vi "Set SPAN Component.vi"(7 "Protocol_only":bool, 8 "error in (no error)":errorcluster caption="Fehler (Eingang, kein Fehler)", 9 "Gasnummer":T3 min=1 max=5, 10 "Autolin Hovacal (alt)":refnum<vi>, 11 "Daten Hovacal (alt)":refnum<vi>) -> (0 "error out":errorcluster caption="Fehler (Ausgang)", 1 "Gaskomponente":T2, 2 "LogInfo-Einstellung-Cluster":T1, 3 "Komponente":string, 4 "Einheit in String":string)   [LabVIEW 2020, in "Linearisierung v2.lvlib" / "SpanEinstellungen.lvlib"]
uses:
  SpanEinstellungen.lvlib
  Gasnumber.ctl
  Visualisierungs Elemente/Auswahlfeld.ctl
  Seiten/FT-IR/FGV FT-IR Gasliste Aktionen.ctl
  Aktion Lin Daten aufarbeiten.ctl
  Gasteiler/Aktionen FGV Gasteiler Daten.ctl
  Linearisierung v2.lvlib
  Seiten/FT-IR/FT-IR.lvlib
  Gasteiler/Gasteiler.lvlib
  Gasteiler/HovaCal/Aktion_FGV_Betriebsdaten.ctl
  Gasteiler/HovaCal/HovaCal.lvlib
  Gasteiler/HovaCAL_Interface/Kommunikation/Kommunikation.lvlib
  Gasteiler/HovaCAL_Interface/Helper/Helper.lvlib
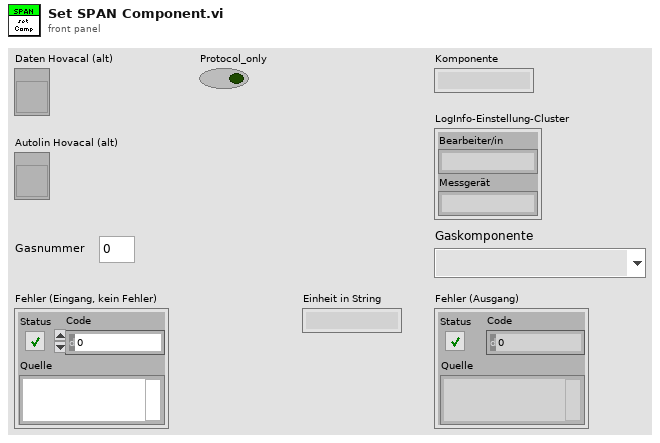
[diagram p1: front panel]
types:
  T1 = cluster{"Bearbeiter/in":string, "Messgerät":string}
  T2 = typedef "Auswahlfeld.ctl" = u16
  T3 = typedef "Linearisierung v2.lvlib/Gasnumber.ctl" = u8
  T4 = typedef "Linearisierung v2.lvlib/Gasteiler.lvlib/Aktionen FGV Gasteiler Daten.ctl" = enum16{"lesen", "Gasteiler Daten", "Seriellen Param.", "MB-Endwert", "laden", "speichern", "Anforderung", "TCP", "Aufzeichnung Start"}
  T5 = typedef "Linearisierung v2.lvlib/Aktion Lin Daten aufarbeiten.ctl" = enum16{"lesen", "Protkolldaten", "speichern", "laden", "EPA auswerten", "Tabelle schreiben", "Lin auswerten", "Tab init", "Stufentabelle", "EPA aktiviert", "Nachbehandlung laden", "Tabelle löschen", "Istwerte löschen", "Zeile löschen", "Zeile einfügen", "LIN aktiviert", "LIN/EPA aktiv laden", "EGAK Tab", "LIN übernehmen", "Tab init ohne Stufen"}
  T6 = typedef "FT-IR.lvlib/FGV FT-IR Gasliste Aktionen.ctl" = enum16{"lesen", "Gasliste FT-IR", "Gasliste ausgelesen", "laden", "speichern", "löschen"}
  T7 = typedef "Linearisierung v2.lvlib/Lin-Polynom Daten.ctl" = cluster{"Messgerät":string, "Kalibrator (Gasteiler)":string, "Bearbeiter/in":string, "Komponente":string, "Zeitstempel":timestamp, "F_max gefordert (%)":sgl, "F_max in %":sgl, "F_max in ppm":sgl, "Vorschlag Ordnung":i32, "Polynom OK":bool, "Polynomkoeff.":dbl[], "Prüfgas Konzentration":dbl, "Pfad EPA":string, "Pfad_LIN":string, "Gasnummer:":u8, "Komponentenauswahl":T8, "Verdünnungsgas":T9, "Zeitdauer Stufe":T10, "Anzahl Stufen":T10, "F_max in % EPA":sgl, "F_max in ppm EPA":sgl, "F_max in % LIN":sgl, "F_max in ppm LIN":sgl, "Punkte umkehren":bool, "EPA Optionsfeld":T11, "Autolin Hovacal":T12, "Spanfactors":sgl[], "Kalibrierauswahl":T13, "Conditions:":T14, "Gasflaschen Nr.:":string, "Bottle Accuracy":dbl, "Konfig Gasflasche":T15, "Gasflasche":T16, "HovaCAL Flow AutoLin":T17, "MFC Output":T18, "Gas Ablaufdatum":timestamp, "Lin Modus":T19, "zusätzliche Zeitdauer Erster Punkt":sgl, "Offsets":sgl[]}
  T8 = typedef "Linearisierung v2.lvlib/KomponentenArray.ctl" = cluster{"Komponente:":T2, "Konzentration":dbl}[]
  T9 = typedef "Linearisierung v2.lvlib/Gasteiler.lvlib/Prüfgas in.ctl" = u16
  T10 = typedef "Zahlen-Eingabefeld.ctl" = sgl
  T11 = typedef "Linearisierung v2.lvlib/EPA Optionsfeld.ctl" = enum32{"Istwert", "Rohwert", "Linearisierter Wert"}
  T12 = typedef "Linearisierung v2.lvlib/Gasteiler.lvlib/HovaCal.lvlib/AutoLin Hovacal.ctl" = enum32{"Keine Auswahl", "Optionsauswahl 1", "Optionsauswahl 2"}
  T13 = typedef "Linearisierung v2.lvlib/Kalibrieroption.ctl" = u16
  T14 = typedef "Linearisierung v2.lvlib/Linearity verification 1065-307.lvlib/Condition.ctl" = u16
  T15 = typedef "System Einstellungen V2.lvlib/Konfig Gasflasche.ctl" = bool
  T16 = typedef "System Einstellungen V2.lvlib/Gasflasche Auswahl.ctl" = u16
  T17 = typedef "Linearisierung v2.lvlib/Gasteiler.lvlib/HovaCAL_Interface.lvlib/Controls.lvlib/Flow Einstellung.ctl" = cluster{"HovaCAL Flow Input Cluster":dbl}
  T18 = typedef "Linearisierung v2.lvlib/Gasteiler.lvlib/HovaCAL_Interface.lvlib/Controls.lvlib/Pump state.ctl" = cluster{"Run":bool}
  T19 = typedef "CalGas Aufschaltung.lvlib/Lin Modus.ctl" = u16
  T20 = typedef "String - Ausgabefeld.ctl" = string
  T21 = typedef "Linearisierung v2.lvlib/Gasteiler.lvlib/HovaCal.lvlib/Aktion_FGV_Betriebsdaten.ctl" = enum16{"Lesen", "Sollwerte schreiben", "Sollwerte lesen", "Gase schreiben", "Gase lesen", "Dynamische Werte", "GaseRef", "Gase aendern"}
  T22 = typedef "Linearisierung v2.lvlib/Gasteiler.lvlib/HovaCal.lvlib/Betriebsdaten.ctl" = cluster{"Gesamtdurchfluss":dbl, "Eingangskonzentration \nTrägergas":dbl, "Eingangskonzentration\nKomponente 1":dbl, "Eingangskonzentration \nKomponente 2":dbl, "Ausgangskonzentration \nKomponente 1 ":dbl, "Ausgangskonzentration\nKomponente 2":dbl, "l/min -> ml/min":bool, "N2 %->ppm":bool, "Komp1 ppm->%":bool, "Komp2ppm->%":bool, "Sollkomp1ppm->%":bool, "Sollkomp2ppm->%":bool}
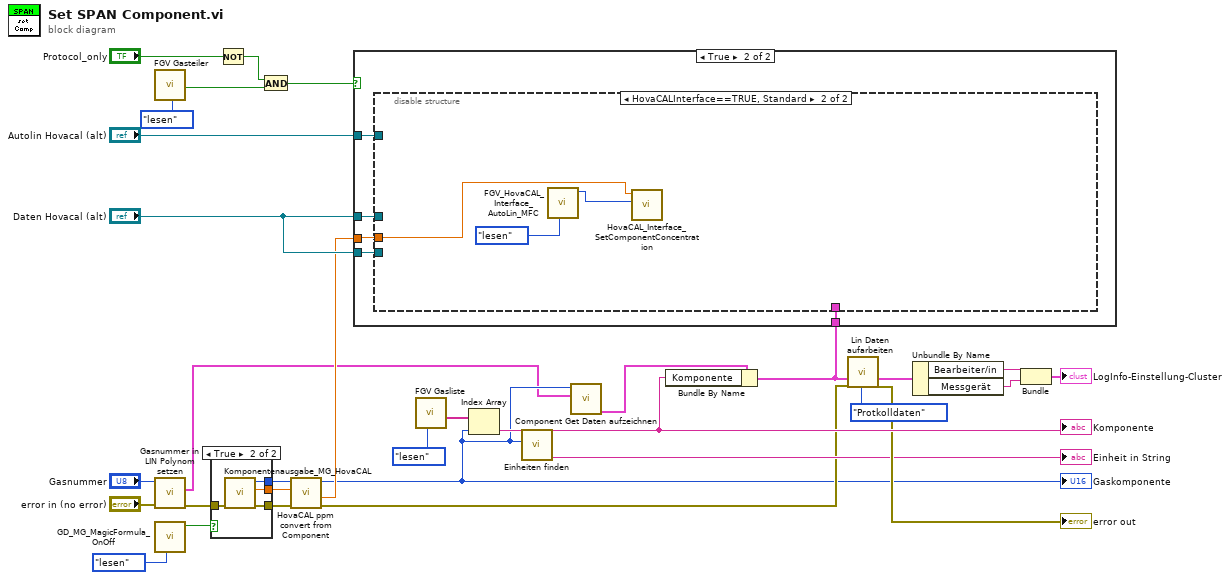
[diagram p0: block diagram]
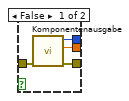
[diagram p2: hidden frame]
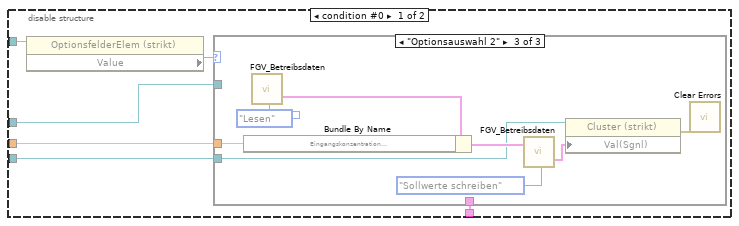
[diagram p4: hidden frame]
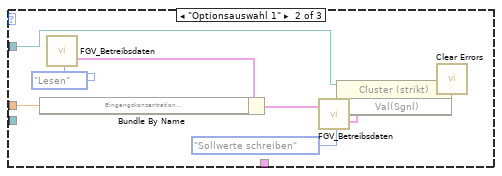
[diagram p6: hidden frame]
diagram:
  n1 = call "FGV Gasteiler.vi"("Aktionen"=Aktionen_FGV_Gasteiler_Daten."lesen") -> ("Anforderung"=w29:bool)  [unwired: 11 in, 7 out]
  n2 = call "Gasnummer in LIN Polynom setzen.vi"("Fehler (Eingang, kein Fehler)"="error in (no error)", "Gasnummer"="Gasnummer") -> ("Fehler (Ausgang)"=w7:errorcluster, "Lin-Polynom"=w2:T7)  [unwired: 7 in, 1 out]
  n3 = call "GD_MG_MagicFormula_OnOff.vi"("Aktion"=enum16{"lesen", "schreiben", "init"}."lesen") -> ("MG_use_magic_formula"=w5:bool)  [unwired: 8 in, 1 out]
  n4 = case shown="True" w5 {
    tunnel: [w33 w38] -> w9
    tunnel: [w34 w37] -> w8
    tunnel: w7 -> [w32 w36]
    tunnel: [w31 w35] -> w6
    frame False {
      n5 = call "Komponentenausgabe.vi"("error in (no error)"=w32) -> ("error out"=w31:errorcluster, "Konzentration"=w33:sgl, "Gaskomponente"=w34:T2)  [unwired: 7 in, 1 out]
    }
    frame True {
      n6 = call "Komponentenausgabe_MG_HovaCAL.vi"("error in (no error)"=w36) -> ("error out"=w35:errorcluster, "GesamtKonzentration"=w38:sgl, "Gaskomponente"=w37:T2)  [unwired: 2 in, 6 out]
    }
  }
  n7 = Not(x="Protocol_only") -> (.not. x?=w12:bool)
  n8 = And(x=w12, y=w29) -> (x .and. y?=w14:bool)
  n9 = call "HovaCAL ppm convert from Component.vi"("Konzentration"=w9, "Gasnummer"=w8) -> ("Konzentration in ppm"=w10:dbl, "Gasnummer out"=w3:T2)  [unwired: 5 in, 3 out]
  "Gaskomponente" <- w3
  n10 = call "FGV Gasliste.vi"("Aktionen"=FGV_FT-IR_Gasliste_Aktionen."lesen") -> ("Aktuelle Gasliste gesamt"=w24:T20[])  [unwired: 8 in, 2 out]
  n11 = Index Array(array=w24, index=w3) -> (element=w26:T20)
  "Komponente" <- w26
  n12 = call "Einheiten finden.vi"("Komponente"=w3) -> ("Einheit in String"=→"Einheit in String":string)  [unwired: 6 in, 4 out]
  n13 = call "Component Get Daten aufzeichnen.vi"("Lin-Polynom"=w2, "Gaskomponente"=w3) -> ("Lin-Polynom out"=w1:T7)  [unwired: 6 in, 3 out]
  n14 = Bundle By Name(cluster=w1, "Komponente"=w26) -> (w27:T7)
  n15 = case shown="True" w14 {
    tunnel: w27 -> [_ w43]
    tunnel: w10 -> [_ w42]
    tunnel: "Daten Hovacal (alt)" -> [_ w41]
    tunnel: "Daten Hovacal (alt)" -> [_ w40]
    tunnel: "Autolin Hovacal (alt)" -> [_ w39]
    frame False {
    }
    frame True {
      n16 = disable-structure shown="HovaCALInterface==TRUE, Standard" {
        disable-tunnel: w43 -> [w49 _]
        disable-tunnel: w42 -> [w48 w66]
        disable-tunnel: w41 -> [w46 _]
        disable-tunnel: w40 -> [w45 _]
        disable-tunnel: w39 -> [w44 _]
        frame condition #0 {
          n17 = property class="OptionsfelderElem (strikt)"(reference=w44) -> ("Value"=w47:T12)  [unwired: 1 in, 2 out]
          n18 = case shown="\"Optionsauswahl 2\"" w47 {
            tunnel: w48 -> [_ w55 w63]
            tunnel: w49 -> [_ _ _]
            tunnel: w46 -> [_ w50 _]
            tunnel: w45 -> [_ _ w58]
            frame "Keine Auswahl", Default {
            }
            frame "Optionsauswahl 1" {
              n19 = call "FGV_Betreibsdaten.vi"("Enum"=Aktion_FGV_Betriebsdaten."Lesen") -> ("Sollwert für Vergleich"=w53:T22)  [unwired: 11 in, 7 out]
              n20 = Bundle By Name(cluster=w53, "Eingangskonzentration\nKomponente 1"=w55) -> (w57:T22)
              n21 = call "FGV_Betreibsdaten.vi"("Sollwert schreiben"=w57, "Enum"=Aktion_FGV_Betriebsdaten."Sollwerte schreiben") -> ("Sollwert für Vergleich"=w54:T22)  [unwired: 10 in, 7 out]
              n22 = property on="Eigenschaftsknoten" class="Cluster (strikt)"(reference=w50, "Val(Sgnl)"=w54) -> (error out=w56:errorcluster)  [unwired: 1 in, 1 out]
              n23 = call <vilib>:"Clear Errors.vi"("error in (no error)"=w56) -> ()  [unwired: 5 in, 2 out]
            }
            frame "Optionsauswahl 2" {
              n24 = call "FGV_Betreibsdaten.vi"("Enum"=Aktion_FGV_Betriebsdaten."Lesen") -> ("Sollwert für Vergleich"=w61:T22)  [unwired: 11 in, 7 out]
              n25 = Bundle By Name(cluster=w61, "Eingangskonzentration \nKomponente 2"=w63) -> (w65:T22)
              n26 = call "FGV_Betreibsdaten.vi"("Sollwert schreiben"=w65, "Enum"=Aktion_FGV_Betriebsdaten."Sollwerte schreiben") -> ("Sollwert für Vergleich"=w62:T22)  [unwired: 10 in, 7 out]
              n27 = property on="Eigenschaftsknoten" class="Cluster (strikt)"(reference=w58, "Val(Sgnl)"=w62) -> (error out=w64:errorcluster)  [unwired: 1 in, 1 out]
              n28 = call <vilib>:"Clear Errors.vi"("error in (no error)"=w64) -> ()  [unwired: 5 in, 2 out]
            }
          }
        }
        frame condition #1 (active) {
          n29 = call "FGV_HovaCAL_Interface_AutoLin_MFC.vi"("Aktion"=enum16{"lesen", "schreiben"}."lesen") -> ("AutoLin MFC out"=w67:u16)  [unwired: 7 in, 3 out]
          n30 = call "HovaCAL_Interface_SetComponentConcentration.vi"("AutoLin MFV Index"=w67, "Konzentration"=w66) -> ()  [unwired: 7 in, 3 out]
        }
      }
    }
  }
  n31 = call "Lin Daten aufarbeiten.vi"("Lin-Polynom"=w27, "error in (no error)"=w6, "Aktionen"=Aktion_Lin_Daten_aufarbeiten."Protkolldaten") -> ("Lin-Polynom"=w18:T7, "error out"=→"error out":errorcluster)  [unwired: 14 in, 9 out]
  n32 = Unbundle By Name(w18) -> ("Bearbeiter/in"=w17:string, "Messgerät"=w16:string)
  n33 = Bundle("Bearbeiter/in"=w17, "Messgerät"=w16) -> (→"LogInfo-Einstellung-Cluster":T1)  [unwired: 1 in]
